vi "Draw Normal.vi"(7 "Auto Defer Panel Updates? (T)":bool=TRUE, 8 "error in (no error)":errorcluster, 11 "Graph Manager in":refnum<class "Graph Manager.lvclass">) -> (0 "error out":errorcluster, 3 "Graph Manager out":refnum<class "Graph Manager.lvclass">)   [LabVIEW 2016, in "Graph Manager.lvclass"]
uses:
  Graph Manager.lvclass
  Graph Manager.lvclass/Graph Manager.ctl
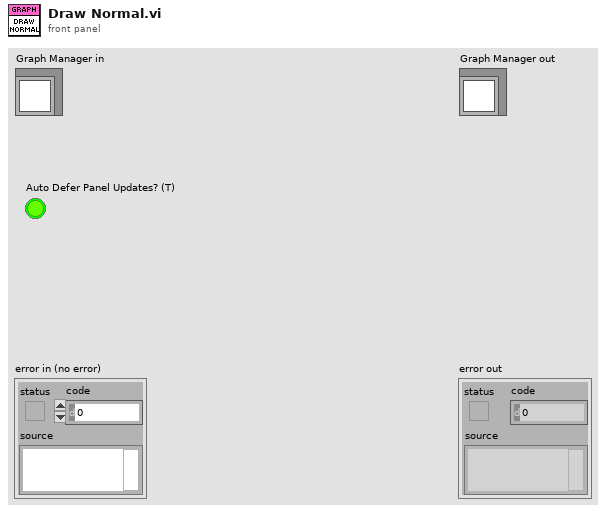
[diagram p1: front panel]
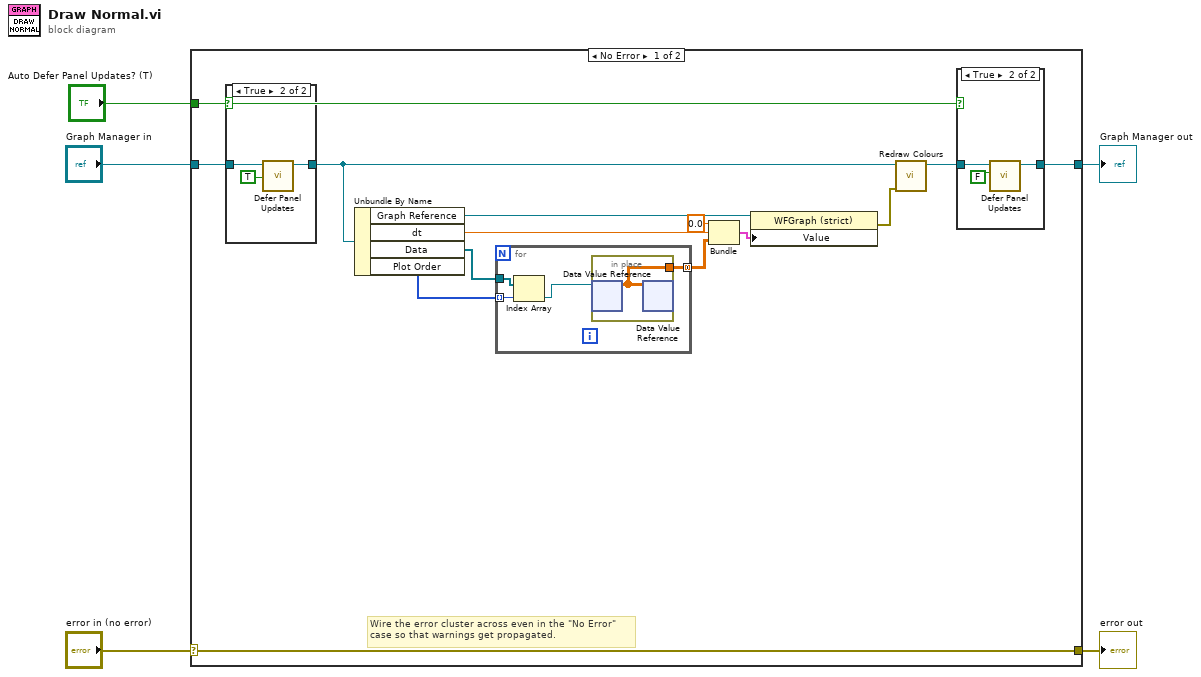
[diagram p0: block diagram]
diagram:
  n1 = case shown="No Error" "error in (no error)" {
    selector: "error in (no error)" -> [w19 w34]
    tunnel: [w19 w34] -> w4
    tunnel: [w15 w33] -> w2
    tunnel: "Graph Manager in" -> [w16 w33]
    tunnel: "Auto Defer Panel Updates? (T)" -> [w6 _]
    frame No Error {
      # "Wire the error cluster across even in the \"No Error\"\ncase so that warnings get propagated."
      n2 = case shown="True" w6 {
        tunnel: [w24 w27] -> w17
        tunnel: w16 -> [w24 w26]
        frame False {
        }
        frame True {
          n3 = call-dynamic "Defer Panel Updates.vi"("Defer Panel Updates"=TRUE, "Graph Manager in"=w26) -> ("Graph Manager out"=w27:refnum<class "Graph Manager.lvclass">)  [unwired: 8 in, 1 out]
        }
      }
      n4 = Unbundle By Name(w17) -> ("Graph Reference"=w14:refnum<vi>, "dt"=w11:dbl, "Data"=w9:refnum<data-value>[], "Plot Order"=w8:i32[])
      n5 = for {
        tunnel: [w31] -> w10 mode=concatenating
        tunnel: w9 -> [w30]
        tunnel: w8 -> [w28] mode=indexing
        n6 = Index Array(array=w30, index=w28) -> (element=w29:refnum<data-value>)
        n7 = in-place {
          in-place-border: [w32] -> w31
          n8 = in-place-dvr #1(w29) -> (w32:dbl[][])  [unwired: 1 out]
          n9 = in-place-dvr #1(w32) -> ()  [unwired: 2 out]
        }
      }
      n10 = Bundle(0.0, "dt"=w11, "Impulse Data"=w10) -> (w13:cluster{dbl, "dt":dbl, "Impulse Data":dbl[][]})  [unwired: 1 in]
      n11 = property class="WFGraph (strict)"(reference=w14, "Value"=w13) -> (error out=w7:errorcluster)  [unwired: 1 in, 1 out]
      n12 = call-dynamic "Redraw Colours.vi"("error in (no error)"=w7, "Graph Manager in"=w17) -> ("Graph Manager out"=w18:refnum<class "Graph Manager.lvclass">)  [unwired: 8 in, 1 out]
      n13 = case shown="True" w6 {
        tunnel: w18 -> [w20 w23]
        tunnel: [w20 w22] -> w15
        frame False {
        }
        frame True {
          n14 = call-dynamic "Defer Panel Updates.vi"("Defer Panel Updates"=FALSE, "Graph Manager in"=w23) -> ("Graph Manager out"=w22:refnum<class "Graph Manager.lvclass">)  [unwired: 8 in, 1 out]
        }
      }
    }
    frame Error {
    }
  }
  "error out" <- w4
  "Graph Manager out" <- w2
